vi "Create All Endpoints as Load.vi"(8 "error in":errorcluster, 10 "topology":string, 11 "endpoint configuration in":T1 format="%.0x") -> (0 "error out":errorcluster, 3 "endpoint configuration out":T1 format="%.0x")   [LabVIEW 2019, in "NI-SWITCH Scripting.lvlib"]
uses:
  NI-SWITCH Scripting.lvlib
  <vilib>/NI VeriStand/Custom Device API/Custom Device Item Ref.ctl
  Shared/Endpoint Configuration Cluster.ctl
  Shared/Endpoint Configuration Enum.ctl
  Shared/NI-SWITCH Shared.lvlib
  <vilib>/NI VeriStand/Custom Device API/Custom Device API.lvlib
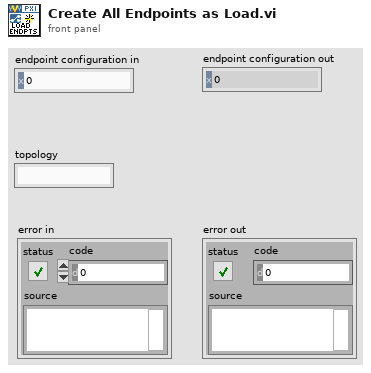
[diagram p1: front panel]
types:
  T1 = typedef "Custom Device API.lvlib/Custom Device Item Ref.ctl" = u64
  T2 = typedef "NI-SWITCH Shared.lvlib/Endpoint Configuration Enum.ctl" = enum16{"Load", "Source", "Configuration"}
  T3 = typedef "NI-SWITCH Shared.lvlib/Endpoint Configuration Cluster.ctl" = cluster{"Endpoint":string, "Configuration":T2}
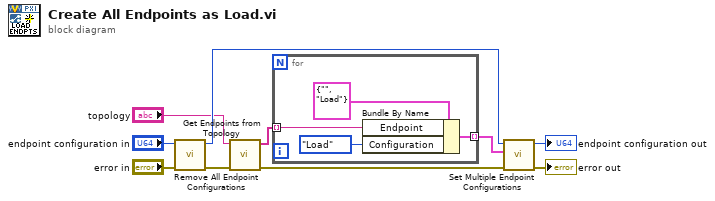
[diagram p0: block diagram]
diagram:
  n1 = call "Remove All Endpoint Configurations.vi"("error in"="error in", "endpoint configuration in"="endpoint configuration in") -> ("error out"=w5:errorcluster, "endpoint configuration out"=w2:T1)  [unwired: 8 in]
  n2 = call "Get Endpoints from Topology.vi"("error in"=w5, "topology"="topology") -> ("error out"=w10:errorcluster, "endpoints"=w7:string[])  [unwired: 8 in]
  n3 = for {
    tunnel: w7 -> [w13] mode=indexing
    tunnel: [w11] -> w6 mode=indexing
    n4 = Bundle By Name(cluster=T3 {"Endpoint"="", "Configuration"=enum."Load"} ("All Endpoint Configurations"), "Endpoint"=w13, "Configuration"=Endpoint_Configuration_Enum."Load") -> (w11:T3)
  }
  n5 = call "Set Multiple Endpoint Configurations.vi"("error in"=w10, "endpoint configurations"=w6, "endpoint configuration in"=w2) -> ("error out"=→"error out":errorcluster, "endpoint configuration out"=→"endpoint configuration out":T1)  [unwired: 7 in]
